vi "find_pipetteTip_v5.vi"(6 "manip position":T3={"width x"=498.0, "height y"=180.0, "x offset"=32.0, "y offset"=116.0}, 7 "slice view":T4, 8 "error in":errorcluster, 9 "pipette match score":sgl=600.0, 10 "pipette template":T4, 11 "pipette in":T1={"Actuator COM"="COM14", "Actuator type"=enum."Scientifica"}) -> (0 "error out":errorcluster, 1 "tip found?":bool, 2 "screen tip location (px)":i32[](array[numeric]), 3 "pipette out":T1={"Actuator COM"="COM14", "Actuator type"=enum."Scientifica"}, 4 "Score":sgl, 5 "found":T4(plugin-control))   [LabVIEW 2015]
uses:
  <vilib>/vision/NI_Vision_Development_Module.lvlib
  <vilib>/vision/Image Controls.llb/IMAQ Image.ctl
  pipette cleaning/pressure box/cleaning_soft/controls/actuator_type.ctl
  pipette cleaning/pressure box/cleaning_soft/controls/actuator_cluster.ctl
panel:
  in  "z moves":i32[](array[numeric])=[0, 10, 10, 10, 10, 10, 10, 10, 10, 10, 10, 10, 10, 10, 10, 10, -150, -10, -10, -10, -10, -10, -10, -10, -10, -10, -10, -10, -10, -10, -10, -10, 150]
  in  "autofocus on?":bool=TRUE
  out "Matches (pixel)":T5(array[cluster]) {"Bounding Box"."y" format="%.2f"; "Bounding Box"."x" format="%.2f"; "Score" format="%.2f"; "Scale" format="%.2f"; "Angle" format="%.2f"; "Position"."y" format="%.2f"; "Position"."x" format="%.2f"}
  out "Number of Matches Found":i32
  in  "Match Parameters":T6={"Number of Matches Requested"=1, "Minimum Match Score"=500.0, "Angle Ranges"=[]} {"Angle Ranges"."End Angle" min=-360 max=360; "Angle Ranges"."Start Angle" min=-360 max=360; "Minimum Match Score" min=0 max=1000; "Number of Matches Requested" min=1 max=9999}
  in  "Algorithm":i32(ring)=1 items=["All", "Low Discrepancy Sampling", "Grayscale Value Pyramid", "Gradients Pyramid"]
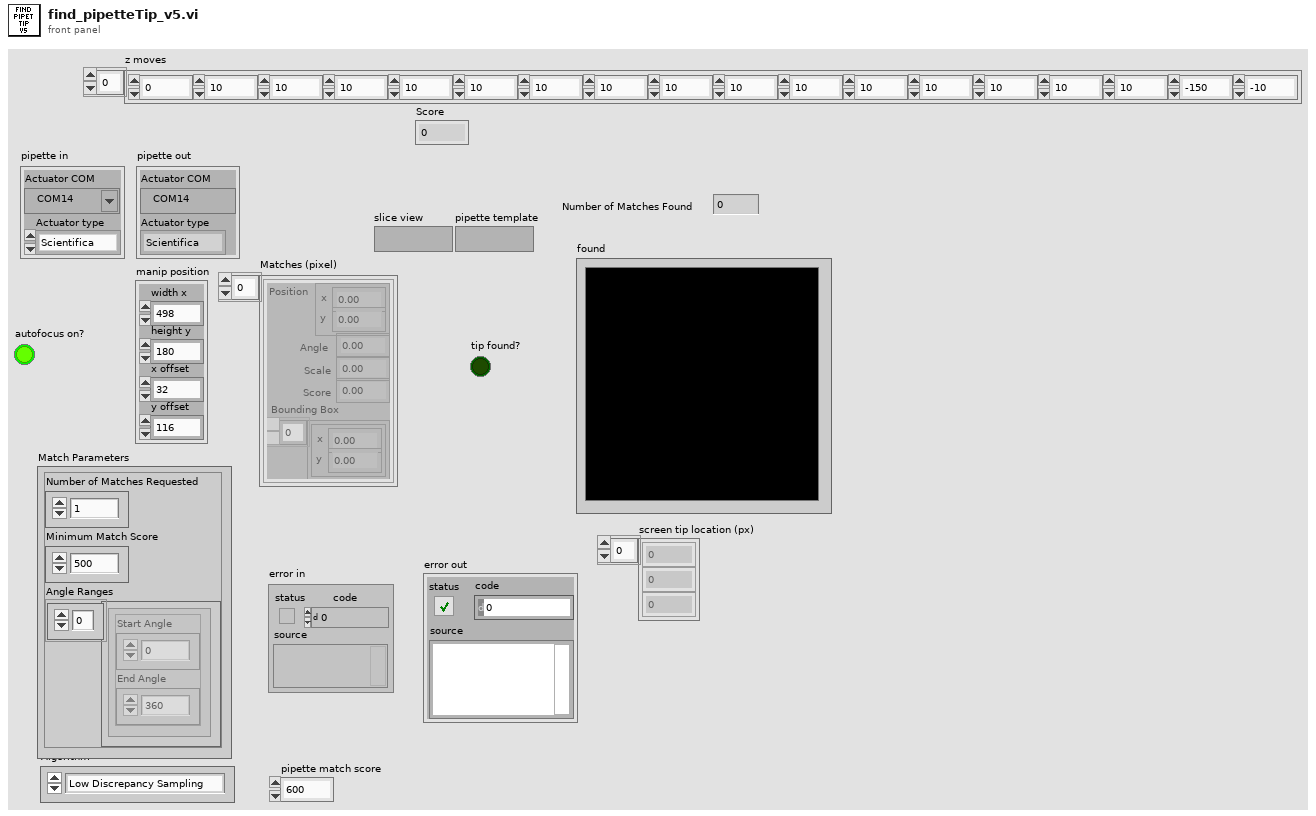
[diagram p1: front panel]
types:
  T1 = typedef "actuator_cluster.ctl" = cluster{"Actuator COM":refnum<visa-resource-name>, "Actuator type":T2}
  T2 = typedef "actuator_type.ctl" = enum16{"Scientifica", "Sutter", "Demo", "Off"}
  T3 = cluster{"width x":dbl, "height y":dbl, "x offset":dbl, "y offset":dbl}
  T4 = typedef "IMAQ Image.ctl" = refnum<image>
  T5 = cluster{"Position":cluster{"x":sgl, "y":sgl}, "Angle":sgl, "Scale":sgl, "Score":sgl, "Bounding Box":cluster{"x":sgl, "y":sgl}[]}[]
  T6 = cluster{"Number of Matches Requested":i32, "Minimum Match Score":sgl, "Angle Ranges":cluster{"Start Angle":sgl, "End Angle":sgl}[]}
  T7 = typedef "Image Type" = u32
  T8 = cluster{"Position":cluster{"x":sgl, "y":sgl}, "Angle":sgl, "Scale":sgl, "Score":sgl, "Bounding Box":cluster{"x":sgl, "y":sgl}[]}
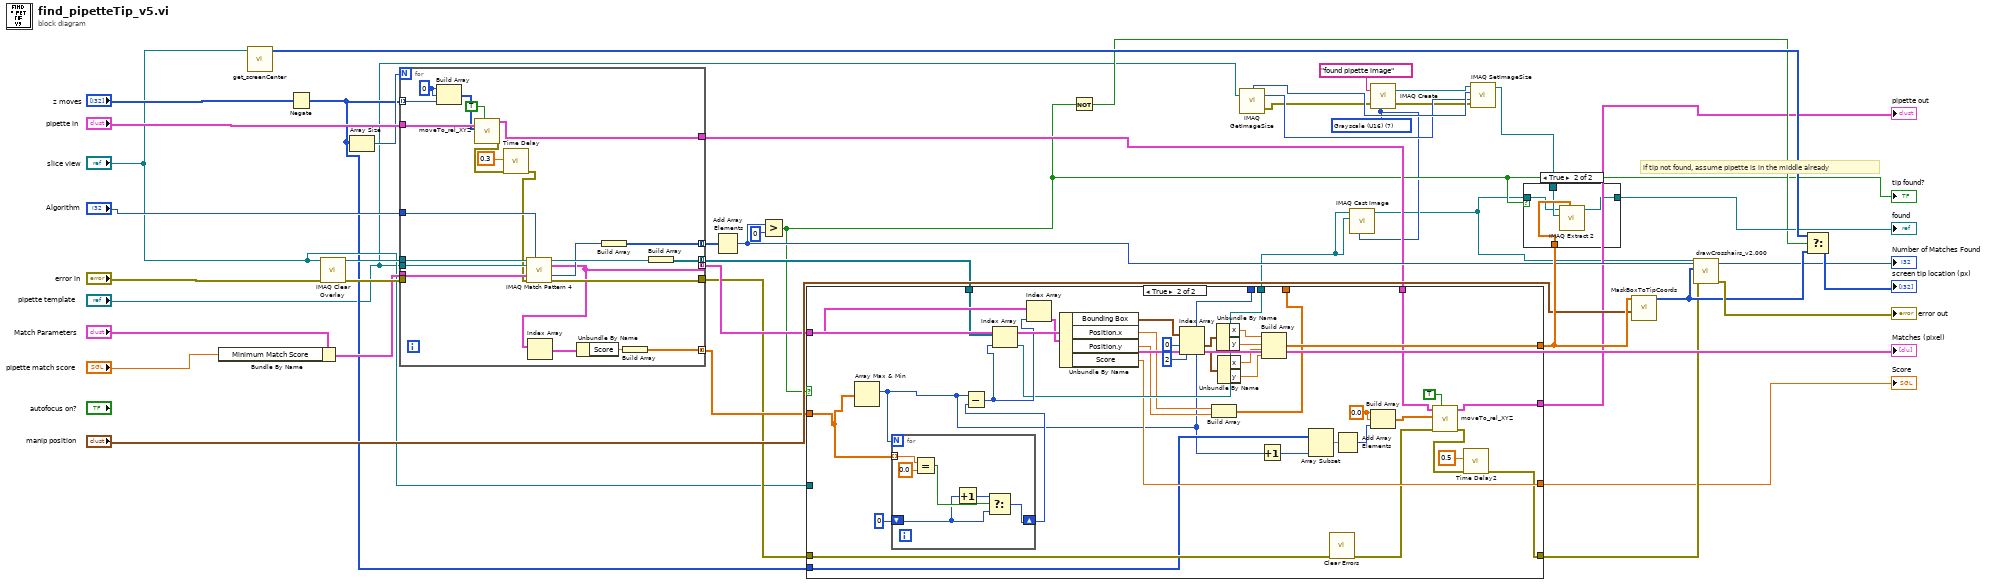
[diagram p0: block diagram]
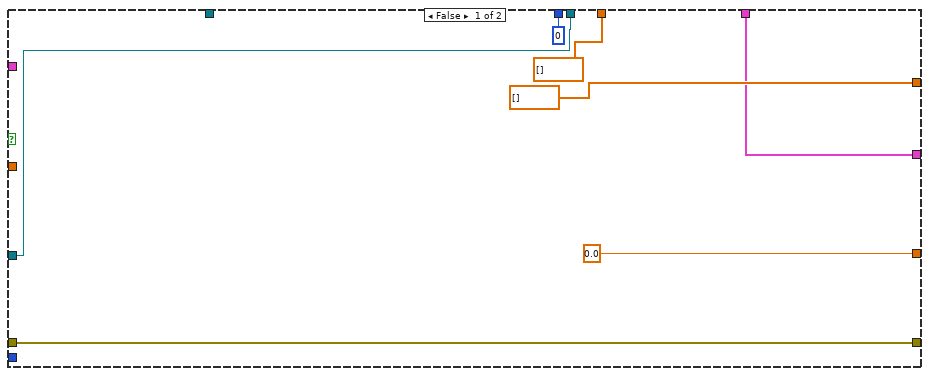
[diagram p3: hidden frame]
diagram:
  w2 = T7 7 items=["Grayscale (U8)", "Grayscale (I16)", "Grayscale (SGL)", "Complex (CSG)", "RGB (U32)", "HSL (U32)", "RGB (U64)", "Grayscale (U16)"] ("Image Type")
  # "if tip not found, assume pipette is in the middle already"
  n1 = Bundle By Name(cluster="Match Parameters", "Minimum Match Score"="pipette match score") -> (w34:T6)
  n2 = call "get_screenCenter.vi"("image"="slice view") -> ("screen center (px)"=w40:i32[])  [unwired: 10 in]
  n3 = Negate(x="z moves") -> (-x=w13:i32[])
  n4 = call "IMAQ Clear Overlay"("error in (no error)"="error in", "Image"="slice view") -> ("error out"=w43:errorcluster, "Image Out"=w29:T4)  [unwired: 8 in]
  n5 = Array Size(array=w13) -> (size(s)=w24:i32)
  n6 = for {
    N: w24 -> [_]
    tunnel: "pipette template" -> [w64]
    tunnel: [w47] -> w23 mode=concatenating
    tunnel: w34 -> [w62]
    tunnel: w29 -> [w65]
    tunnel: [w45] -> w17 mode=concatenating
    tunnel: w43 -> [_]
    tunnel: [w61] -> w19
    tunnel: "pipette in" -> [w60]
    tunnel: w13 -> [w59] mode=indexing
    tunnel: [w56] -> w14
    tunnel: "Algorithm" -> [w54]
    tunnel: [w46] -> w26 mode=concatenating
    tunnel: [w44] -> w20 mode=concatenating
    w58 = 0 ("element")
    n7 = Build Array(w58, w58, w59) -> (w57:i32[])
    n8 = call "moveTo_rel_XYZ.vi"("blocking?"=TRUE, "XYZ location (steps)"=w57, "Actuator cluster in"=w60) -> ("error out"=w49:errorcluster, "Actuator cluster out"=w56:T1)  [unwired: 7 in]
    n9 = call "Time Delay"("error in (no error)"=w49, "Delay Time (s)"=0.3) -> ("error out"=w48:errorcluster)  [unwired: 9 in]
    n10 = call "IMAQ Match Pattern 4"("Image"=w65, "Algorithm"=w54, "Template Image"=w64, "Parameters"=w62, "error in (no error)"=w48) -> ("Image (duplicate)"=w63:T4, "Matches (pixel)"=w47:T5, "Number of Matches"=w53:i32, "error out"=w61:errorcluster)  [unwired: 6 in, 1 out]
    n11 = Index Array(array=w47) -> (element=w55:T8)  [unwired: 1 in]
    n12 = Unbundle By Name(w55) -> ("Score"=w52:sgl)
    n13 = Build Array(w53) -> (w46:i32[])
    n14 = Build Array(w52) -> (w44:sgl[])
    n15 = Build Array(w63) -> (w45:T4[])
  }
  "Matches (pixel)" <- w23
  n16 = Add Array Elements(numeric array=w26) -> (sum=w22:i32)
  "Number of Matches Found" <- w22
  n17 = Greater?(x=w22, y=0) -> (0:w11:bool)
  "tip found?" <- w11
  n18 = case shown="True" w11 {
    tunnel: [sgl[] [] w99] -> w37
    tunnel: w23 -> [_ w98]
    tunnel: w20 -> [_ w95]
    tunnel: w19 -> [w68 w78]
    tunnel: [w68 w79] -> w18
    tunnel: w17 -> [_ w94]
    tunnel: [0 w76] -> _
    tunnel: [w67 w92] -> w3
    tunnel: [sgl[] [] w89] -> _
    tunnel: [sgl 0.0 ("Score") w88] -> w15
    tunnel: "slice view" -> [w67 _]
    tunnel: w14 -> [w66 w83]
    tunnel: w13 -> [_ w77]
    tunnel: [w66 w74] -> w12
    frame False {
    }
    frame True {
      w81 = 0.0 ("element")
      n19 = Array Max & Min(array=w95) -> (max index (indices)=w76:i32)  [unwired: 3 out]
      n20 = for {
        N: w76 -> [_]
        tunnel: w95 -> [w115] mode=indexing
        shift-right: [w110] -> w96
        shift-left: 0 -> [w112]
        n21 = Equal?(x=w115, y=sgl 0.0) -> (x = y?=w113:bool)
        n22 = Increment(x=w112) -> (x+1=w111:i32)
        n23 = Select(t=w111, s=w113, f=w112) -> (s? t:f=w110:i32)
      }
      n24 = Subtract(x=w76, y=w96) -> (x-y=w93:i32)
      n25 = Index Array(array=w94, index=w93) -> (element=w92:T4)
      n26 = Index Array(array=w98, index=w93) -> (element=w109:T8)
      n27 = Unbundle By Name(w109) -> ("Bounding Box"=w108:cluster{"x":sgl, "y":sgl}[], "Position.x"=w91:sgl, "Position.y"=w90:sgl, "Score"=w88:sgl)
      n28 = Index Array(array=w108, index #1=0 ("index"), index #2=2 ("index")) -> (element #1=w105:cluster{"x":sgl, "y":sgl}, element #2=w104:cluster{"x":sgl, "y":sgl})
      n29 = Build Array(w91, w90) -> (w89:sgl[])
      n30 = Unbundle By Name(w105) -> ("x"=w101:sgl, "y"=w100:sgl)
      n31 = Unbundle By Name(w104) -> ("x"=w103:sgl, "y"=w102:sgl)
      n32 = Increment(x=w76) -> (x+1=w75:i32)
      n33 = Build Array(w101, w100, w103, w102) -> (w99:sgl[])
      n34 = Array Subset(array=w77, length=w75) -> (w87:i32[])  [unwired: 1 in]
      n35 = call <vilib>:"Clear Errors.vi"("error in (no error)"=w78) -> ("error out"=w73:errorcluster)  [unwired: 5 in, 1 out]
      n36 = Add Array Elements(numeric array=w87) -> (sum=w82:i32)
      n37 = Build Array(w81, w81, w82) -> (w80:dbl[])
      n38 = call "moveTo_rel_XYZ.vi"("blocking?"=TRUE, "error in"=w73, "XYZ location (steps)"=w80, "Actuator cluster in"=w83) -> ("error out"=w84:errorcluster, "Actuator cluster out"=w74:T1)  [unwired: 6 in]
      n39 = call "Time Delay2"("error in (no error)"=w84, "Delay Time (s)"=0.5) -> ("error out"=w79:errorcluster)  [unwired: 9 in]
    }
  }
  "pipette out" <- w12
  "Score" <- w15
  n40 = Not(x=w11) -> (.not. x?=w30:bool)
  n41 = call "IMAQ GetImageSize"("Image"="pipette template") -> ("Y Resolution"=w6:i32, "X Resolution"=w7:i32, "error out"=w5:errorcluster)  [unwired: 3 in]
  n42 = call "IMAQ Cast Image"("Image Type"=w2, "Image Dst"=w3, "Image Src"=w3) -> ("Image Dst Out"=w1:T4)  [unwired: 7 in, 1 out]
  n43 = call "IMAQ Create"("Image Name"="found pipette image", "Image Type"=w2, "error in (no error)"=w5) -> ("New Image"=w9:T4, "error out"=w4:errorcluster)  [unwired: 2 in]
  n44 = call "IMAQ SetImageSize"("error in (no error)"=w4, "Y Resolution"=w6, "X Resolution"=w7, "Image"=w9) -> ("Image Out"=w8:T4)  [unwired: 1 in, 1 out]
  n45 = case shown="True" w11 {
    tunnel: w37 -> [_ w120]
    tunnel: [w116 w119] -> w36
    tunnel: w8 -> [w116 w118]
    tunnel: w1 -> [_ w117]
    frame False {
    }
    frame True {
      n46 = call "IMAQ Extract 2"("Optional Rectangle"=w120, "Image Dst"=w118, "Image Src"=w117) -> ("Image Dst Out"=w119:T4)  [unwired: 7 in, 1 out]
    }
  }
  "found" <- w36
  n47 = call "MaskBoxToTipCoords.vi"("manip 1 position"="manip position", "bounding rectangle"=w37) -> ("user selected pipette tip (x,y)"=w39:i32[])  [unwired: 9 in]
  n48 = call "drawCrosshairs_v2.000.vi"("error in (no error)"=w18, "pipette tip location (px)"=w39, "image in"=w1) -> ("error out"=→"error out":errorcluster)  [unwired: 7 in, 1 out]
  n49 = Select(t=w40, s=w30, f=w39) -> (s? t:f=→"screen tip location (px)":i32[])
